vi "_Write.vi"(7 "Message ID":string, 8 "error in (no error)":errorcluster, 10 "Data":string, 11 "StringStream in":refnum<class "StringStream.lvclass">) -> (0 "error out":errorcluster, 3 "StringStream out":refnum<class "StringStream.lvclass">)   [LabVIEW 2020, in "Stream.lvlib" / "StringStream.lvclass"]
uses:
  StringStream.lvclass
  StringStream.lvclass/StringStream.ctl
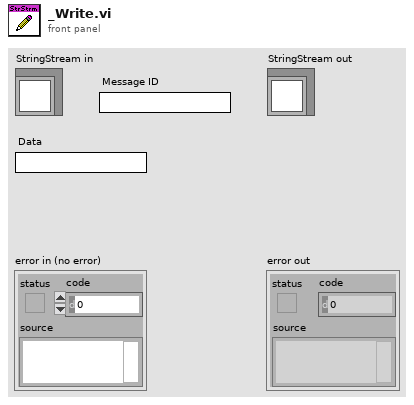
[diagram p1: front panel]
types:
  T1 = typedef "Stream.lvlib/StringStream.lvclass/Ref Data.ctl" = cluster{"Position":i64, "String":string}
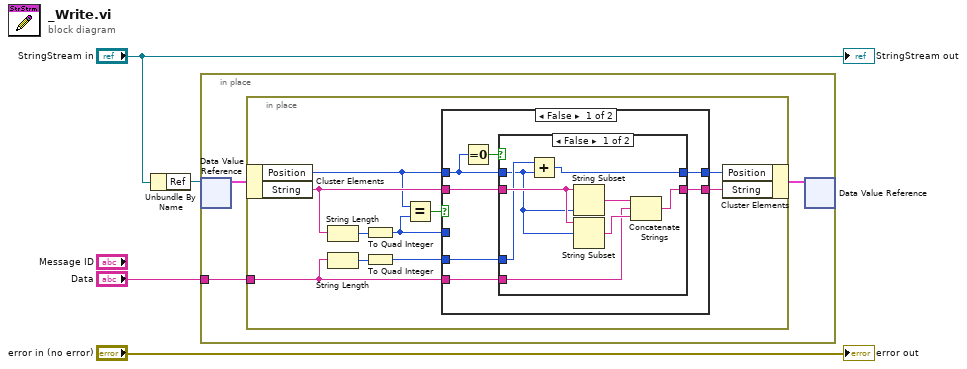
[diagram p0: block diagram]
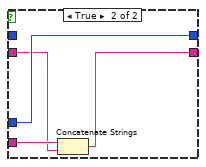
[diagram p2: hidden frame]
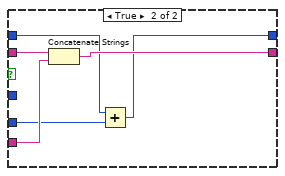
[diagram p3: hidden frame]
diagram:
  n1 = Unbundle By Name("StringStream in") -> ("Ref"=w3:refnum<data-value>)
  n2 = in-place {
    in-place-border: "Data" -> [w5]
    n3 = in-place-dvr #1(w3) -> (w7:T1)  [unwired: 1 out]
    n4 = in-place {
      in-place-border: w5 -> [w10]
      n5 = in-place-cluster #2(w7) -> ("Position"=w12:i64, "String"=w14:string)
      n6 = String Length(string=w14) -> (length=w16:i32)
      n7 = String Length(string=w10) -> (length=w17:i32)
      n8 = To Quad Integer(1:w16) -> (0:w13:i64)
      n9 = To Quad Integer(1:w17) -> (0:w11:i64)
      n10 = Equal?(x=w12, y=w13) -> (x = y?=w15:bool)
      n11 = case shown="False" w15 {
        tunnel: w14 -> [w20 w42]
        tunnel: w13 -> [_ _]
        tunnel: w12 -> [w23 w38]
        tunnel: w11 -> [w22 w39]
        tunnel: w10 -> [w19 w41]
        tunnel: [w18 w40] -> w9
        tunnel: [w21 w37] -> w8
        frame False {
          n12 = Equal To 0?(x=w23) -> (x = 0?=w24:bool)
          n13 = case shown="False" w24 {
            tunnel: w23 -> [w25 _]
            tunnel: w22 -> [w27 w36]
            tunnel: [w26 w36] -> w21
            tunnel: w20 -> [w32 w34]
            tunnel: w19 -> [w29 w35]
            tunnel: [w28 w33] -> w18
            frame False {
              n14 = Add(x=w27, y=w25) -> (x+y=w26:i64)
              n15 = String Subset(string=w32, length (rest)=w25) -> (substring=w31:string)  [unwired: 1 in]
              n16 = String Subset(string=w32, offset (0)=w25) -> (substring=w30:string)  [unwired: 1 in]
              n17 = Concatenate Strings(w31, w29, w30) -> (w28:string)
            }
            frame True {
              n18 = Concatenate Strings(w35, w34) -> (w33:string)
            }
          }
        }
        frame True {
          n19 = Concatenate Strings(w42, w41) -> (w40:string)
          n20 = Add(x=w38, y=w39) -> (x+y=w37:i64)
        }
      }
      n21 = in-place-cluster #2("Position"=w8, "String"=w9) -> (w6:T1)
    }
    n22 = in-place-dvr #1(w6) -> ()  [unwired: 2 out]
  }
  "error out" <- "error in (no error)"
  "StringStream out" <- "StringStream in"
